vi "8.8.4_알림자.vi"() -> ()   [LabVIEW 2018]
panel:
  in  "stop":bool
  in  "test":bool
  out "받은 데이터":string
  in  "보낼 데이터":string
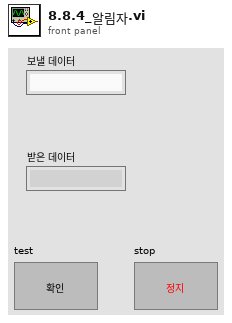
[diagram p1: front panel]
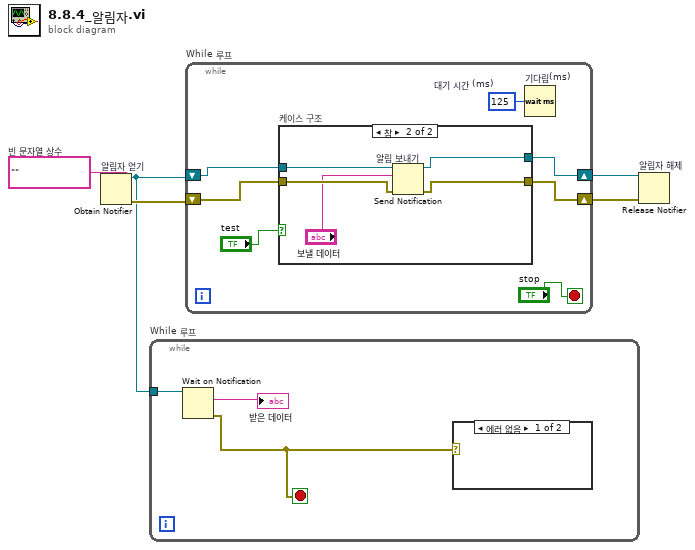
[diagram p0: block diagram]
diagram:
  w2 = ""  # 빈 문자열 상수
  n1 = Obtain Notifier "알림자 얻기"(notification data type=w2) -> (notifier out=w1:refnum<notifier>, error out=w4:errorcluster)  [unwired: 3 in, 1 out]
  n2 = while "While 루프" {
    tunnel: w1 -> [w8]
    stop <- w6 stop-if-true
    n3 = Wait on Notification(notifier=w8) -> (notification=→"받은 데이터":string, error out=w6:errorcluster)  [unwired: 3 in, 2 out]
    n4 = case shown="에러 없음" w6 {
      frame No Error {
      }
      frame Error {
      }
    }
  }
  n5 = while "While 루프" {
    shift-right: [w14] -> w5
    shift-left: w1 -> [w15]
    shift-right: [w12] -> w3
    shift-left: w4 -> [w13]
    stop <- "stop" stop-if-true
    w11 = u32 125  # 대기 시간 (ms)
    n6 = case "케이스 구조" shown="참" "test" {
      tunnel: w15 -> [w17 w22]
      tunnel: [w17 w21] -> w14
      tunnel: w13 -> [w16 w20]
      tunnel: [w16 w19] -> w12
      frame False {
      }
      frame True {
        n7 = Send Notification "알림 보내기"(notification="보낼 데이터", notifier=w22, error in (no error)=w20) -> (notifier out=w21:refnum<notifier>, error out=w19:errorcluster)
      }
    }
    n8 = Wait (ms) "기다림(ms)"(milliseconds to wait=w11) -> ()  [unwired: 1 out]
  }
  n9 = Release Notifier "알림자 해제"(notifier=w5, error in (no error)=w3) -> ()  [unwired: 1 in, 3 out]
